vi "Shoot Select Mode.vi"() -> (3 "Auton Shooter Command":T1={"Shooter Mode"=enum."Disabled", "Throttle (%)/ Vision-based\nSetpoint (RPM)"=0.0, "Shooter Preset speeds (RPM)"=enum."Target Zone", "Timestamp (ms)"=0.0})   [LabVIEW 2019]
uses:
  Shooter Command Type Def.ctl
  Shooter Mode Type Def.ctl
  Shooter Preset speeds Type Def.ctl
  .Team Code/Robot Global Data.vi
  Shoot Global.vi
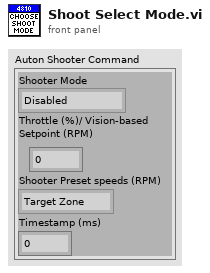
[diagram p1: front panel]
types:
  T1 = typedef "Shooter Command Type Def.ctl" = cluster{"Shooter Mode":T2, "Throttle (%)/ Vision-based\nSetpoint (RPM)":dbl, "Shooter Preset speeds (RPM)":T3, "Timestamp (ms)":dbl}
  T2 = typedef "Shooter Mode Type Def.ctl" = enum16{"Disabled", "Raw Throttle", "Preset Velocity Control", "Vision-based Velocity Control"}
  T3 = typedef "Shooter Preset speeds Type Def.ctl" = enum16{"Not Applicable", "Target Zone", "Initiation Line", "Close end of Trench Run", "Control Panel"}
  T4 = typedef "WPI_DriverStationRobotMode2.ctl" = enum16{"Autonomous Disabled", "Autonomous Enabled", "Teleop Disabled", "Teleop Enabled", "Disconnected", "Finish", "Test Disabled", "Test Enabled", "Emergency Stopped"}
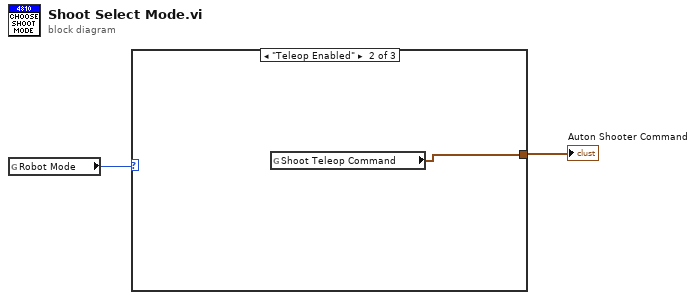
[diagram p0: block diagram]
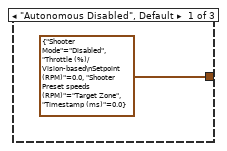
[diagram p2: hidden frame]
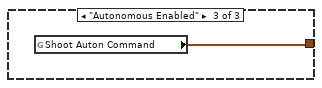
[diagram p3: hidden frame]
diagram:
  n1 = global read "Robot Global Data.vi" "Robot Mode"() -> (w2:T4)
  n2 = case shown="\"Teleop Enabled\"" w2 {
    tunnel: [T1 {"Shooter Mode"=enum."Disabled", "Throttle (%)/ Vision-based\nSetpoint (RPM)"=0.0, "Shooter Preset speeds (RPM)"=enum."Target Zone", "Timestamp (ms)"=0.0} ("Teleop Shooter Command") w4 w5] -> w1
    frame "Autonomous Disabled", Default {
    }
    frame "Teleop Enabled" {
      n3 = global read "Shoot Global.vi" "Shoot Teleop Command"() -> (w4:T1)
    }
    frame "Autonomous Enabled" {
      n4 = global read "Shoot Global.vi" "Shoot Auton Command"() -> (w5:T1)
    }
  }
  "Auton Shooter Command" <- w1
